vi "Manual Scale.vi"(8 "error in (no error)":errorcluster, 9 "Secs/div":dbl, 10 "V/div":T1, 11 "PicoScope 3000a in":refnum<class "PicoScope 3000a.lvclass">) -> (0 "error out":errorcluster, 3 "PicoScope 3000a out":refnum<class "PicoScope 3000a.lvclass">)   [LabVIEW 2018, in "PicoScope 3000a.lvlib" / "PicoScope 3000a.lvclass"]
doc: "This Overrride is used to manually adjust the scale of the instrument. This Overrides needs"
uses:
  PicoScope 3000a.lvclass
  LWS SLA-070/Distro/Projects/12170 Luminar LWS Base/Source/PPLs/Oscilloscope.lvlibp/Custom Controls/Volts per Division.ctl
  LWS SLA-070/Distro/Projects/12170 Luminar LWS Base/Source/PPLs/Oscilloscope.lvlibp/Custom Controls/Analog Channels.ctl
  PicoScope 3000a.lvclass/PicoScope 3000a.ctl
  <instrlib>/PicoScope/PicoScope.lvlib
  LWS SLA-070/Distro/Projects/12170 Luminar LWS Base/Source/PPLs/Oscilloscope.lvlibp
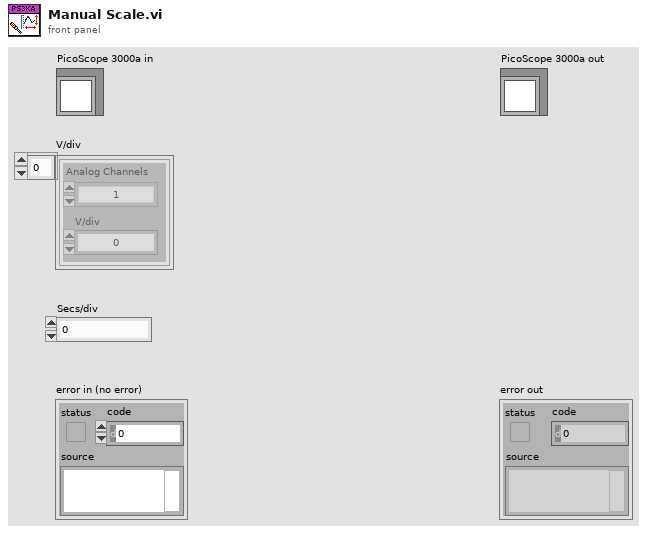
[diagram p1: front panel]
types:
  T1 = typedef "Oscilloscope.lvlibp/Volts per Division.ctl" = cluster{"Analog Channels":T2, "V/div":dbl}[]
  T2 = typedef "Oscilloscope.lvlibp/Analog Channels.ctl" = enum16{"1", "2", "3", "4", "5", "6", "7", "8", "9", "10", "11", "12", "13", "14", "15", "16"}
  T3 = cluster{"Enabled":bool, "Coupling":u32, "Range":u32, "Analogue Offset":sgl}[]
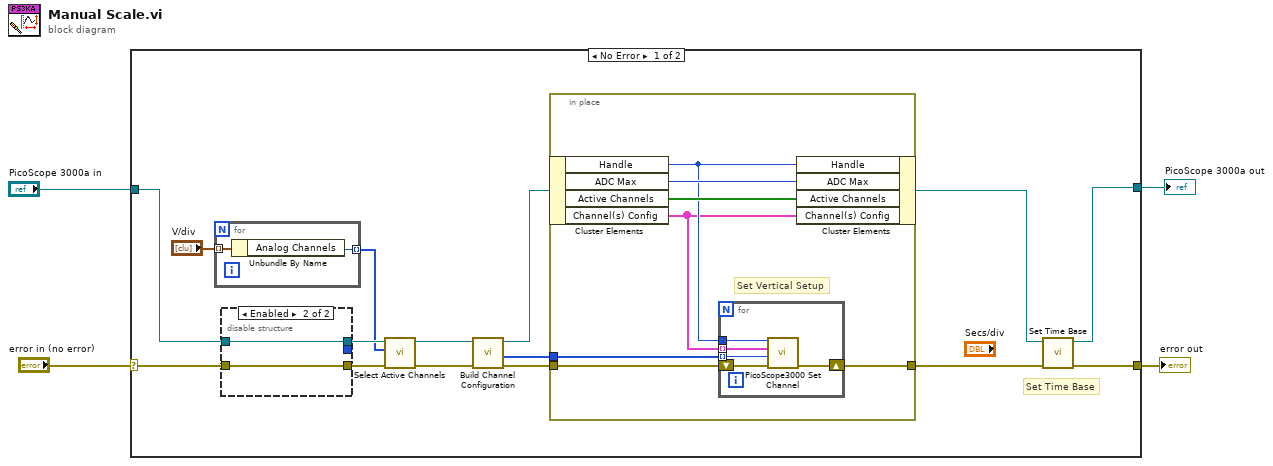
[diagram p0: block diagram]
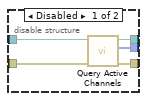
[diagram p2: hidden frame]
diagram:
  n1 = case shown="No Error" "error in (no error)" {
    selector: "error in (no error)" -> [w9 w42]
    tunnel: "PicoScope 3000a in" -> [w10 w41]
    tunnel: [w14 w42] -> w2
    tunnel: [w13 w41] -> w1
    frame No Error {
      # "Set Time Base"
      n2 = for {
        tunnel: "V/div" -> [w21] mode=indexing
        tunnel: [w20] -> w5 mode=indexing
        n3 = Unbundle By Name(w21) -> ("Analog Channels"=w20:T2)
      }
      n4 = disable-structure shown="Enabled" {
        disable-tunnel: [w26 w28] -> w12
        disable-tunnel: [w25 w27] -> w11
        disable-tunnel: [w24 _] -> _
        disable-tunnel: w10 -> [w23 w28]
        disable-tunnel: w9 -> [w22 w27]
        frame Disabled {
          n5 = call "Query Active Channels.vi"("error in (no error)"=w22, "PicoScope 3000a in"=w23) -> ("error out"=w25:errorcluster, "Active Channel(s)"=w24:T2[], "PicoScope 3000a out"=w26:refnum<class "PicoScope 3000a.lvclass">)  [unwired: 7 in]
        }
        frame Enabled {
        }
      }
      n6 = call-dynamic "Select Active Channels.vi"("error in (no error)"=w11, "Active Channel(s)"=w5, "PicoScope 3000a in"=w12) -> ("error out"=w8:errorcluster, "PicoScope 3000a out"=w7:refnum<class "PicoScope 3000a.lvclass">)  [unwired: 7 in]
      n7 = call "Build Channel Configuration.vi"("error in (no error)"=w8, "PicoScope 3000a in"=w7) -> ("error out"=w19:errorcluster, "Channel Numbers"=w17:u32[], "PicoScope 3000a out"=w18:refnum<class "PicoScope 3000a.lvclass">)  [unwired: 7 in]
      n8 = in-place {
        in-place-border: w19 -> [w34]
        in-place-border: w17 -> [w30]
        in-place-border: [w31] -> w16
        # "Set Vertical Setup"
        n9 = in-place-cluster #1(w18) -> ("Handle"=w32:i16, "ADC Max"=w35:i16, "Active Channels"=w33:bool[], "Channel(s) Config"=w29:T3)
        n10 = for {
          tunnel: w29 -> [w38] mode=indexing
          tunnel: w32 -> [w39]
          shift-right: [w37] -> w31
          shift-left: w34 -> [w40]
          tunnel: w30 -> [w36] mode=indexing
          n11 = call <instrlib>:"PicoScope3000 Set Channel.vi"("error in (no error)"=w40, "Channel Settings"=w38, "Channel"=w36, "Handle"=w39) -> ("error out"=w37:errorcluster)  [unwired: 5 in, 2 out]
        }
        n12 = in-place-cluster #1("Handle"=w32, "ADC Max"=w35, "Active Channels"=w33, "Channel(s) Config"=w29) -> (w15:refnum<class "PicoScope 3000a.lvclass">)
      }
      n13 = call "Set Time Base.vi"("error in (no error)"=w16, "PicoScope 3000a in"=w15) -> ("error out"=w14:errorcluster, "PicoScope 3000a out"=w13:refnum<class "PicoScope 3000a.lvclass">)  [unwired: 8 in]
    }
    frame Error {
    }
  }
  "error out" <- w2
  "PicoScope 3000a out" <- w1
